vi "accept signal.vi"() -> ()   [LabVIEW 2019]
panel:
  out "Numeric":dbl
  out "Waveform Graph":waveform(dbl)(graph)
  in  "stop (F)":bool
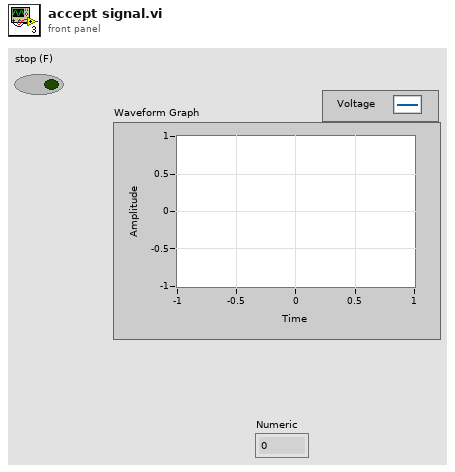
[diagram p1: front panel]
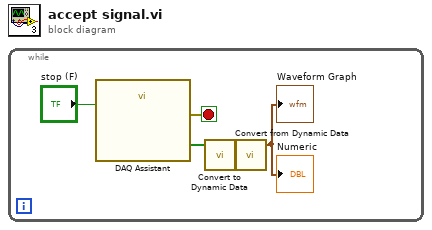
[diagram p0: block diagram]
diagram:
  n1 = while {
    stop <- w4 stop-if-true
    n2 = call "DAQ Assistant"("stop (T)"="stop (F)") -> ("data"=w2:bool[], "error out"=w4:errorcluster)  [unwired: 16 in, 1 out]
    n3 = call "Convert to Dynamic Data"("Array"=w2) -> ("Dynamic Data Type"=w1:dynamicdata)  [unwired: 3 in]
    n4 = call "Convert from Dynamic Data"("Dynamic Data Type"=w1) -> ("Waveform"=→"Waveform Graph" →"Numeric":waveform(dbl))  [unwired: 3 in]
  }
